vi "LSMcontroller_v62_updatedpointscan.vi"() -> ()   [LabVIEW 2015] (continued)
                n4196 = call "waveformsDObuffer.vi"("DO wf in"=w1149, "command"="set") -> ()  [unwired: 1 out]
                n4197 = call "waveformsAObuffer.vi"("AO wf in"=w1151, "command"="set") -> ()  [unwired: 1 out]
                n4198 = local write "Total Camera Frames"(w1150) -> ()
                n4199 = case shown="True" w1147 {
                  tunnel: w1146 -> [_ w1160]
                  frame False {
                  }
                  frame True {
                    n4200 = local write "# of frames"(w1160) -> ()
                  }
                }
              }
              frame #3 {
                n4201 = local read "finite samples"() -> (w1161:bool)
                n4202 = local read "continuous"() -> (w1162:bool)
                n4203 = local read "wavdet"() -> (w1163:bool)
                n4204 = call "2pparameters.vi"("command"="get") -> ("params out"=w1166:T10)  [unwired: 1 in]
                n4205 = Bundle By Name(cluster=w1166, "finite"=w1161, "cont"=w1162, "wavdet"=w1163) -> (w1164:T10)
                n4206 = call "2pparameters.vi"("Params in"=w1164, "command"="set") -> ()  [unwired: 1 out]
              }
            }
          }
          event "Start amplitude (V)", "Cycles", "Baseline (V)", "Step size (V)", "DC (%)", "Period (ms)", "Repeats", "Pulses", "phase shift (ms)": Value Change {
            n4207 = event-data() -> ()  [unwired: 1 in, 6 out]
            n4208 = stacked-sequence {
              seq-local: [_ _ w1274 _ _] -> [_ _ _ w1296 _]
              seq-local: [_ _ w1273 _ _] -> [_ _ _ w1295 _]
              frame #0 {
                n4209 = local read "Measurement"() -> (w1168:T4)
                n4210 = case shown="\"X-Y-t movie\", Default" w1168 {
                  frame "X-Y-t movie", Default {
                    n4211 = local read "avpp"() -> (w1189:i32)
                    n4212 = local read "Angle ref"() -> (w1188:dbl)
                    n4213 = local read "ROI Type"() -> (w1187:u16)
                    n4214 = local read "xpixels ref"() -> (w1184:i32)
                    n4215 = local read "Vx-min ref"() -> (w1183:dbl)
                    n4216 = local read "Vx-max ref"() -> (w1182:dbl)
                    n4217 = local read "ypixels ref"() -> (w1180:i32)
                    n4218 = local read "Vy-min ref"() -> (w1181:dbl)
                    n4219 = local read "Vy-max ref"() -> (w1177:dbl)
                    n4220 = local read "Sampling rate"() -> (w1171:dbl)
                    n4221 = local read "finite samples"() -> (w1172:bool)
                    n4222 = local read "continuous"() -> (w1175:bool)
                    n4223 = local read "wavdet"() -> (w1176:bool)
                    n4224 = local read "# of frames"() -> (w1174:i32)
                    n4225 = local read "maxbufferAI"() -> (w1173:i32)
                    n4226 = local read "Override AI buffer"() -> (w1169:bool)
                    n4227 = call "2pparameters.vi"("command"="get") -> ("params out"=w1186:T10)  [unwired: 1 in]
                    n4228 = Bundle By Name(cluster=w1186, "type"="X-Y-t movie", "avpp"=w1189, "Angle Img"=w1188, "Xpixels Img"=w1184, "Vx-min Img"=w1183, "VX-max Img"=w1182, "Ypixels Img"=w1180, "Vy-min Img"=w1181, "Vy-max Img"=w1177, "srate"=w1171, "srate Img"=w1171, "finite"=w1172, "cont"=w1175, "wavdet"=w1176, "measpoints"=w1174, "maxbufferAI"=w1173, "Drawing Mode"=w1187, "Vz-reset"=0.0, "AIoverride"=w1169) -> (w1178:T10)
                    n4229 = call "2pparameters.vi"("Params in"=w1178, "command"="set") -> ()  [unwired: 1 out]
                  }
                  frame "X-Y-Z stack" {
                    n4230 = call "2pparameters.vi"("command"="get") -> ("params out"=w1193:T10)  [unwired: 1 in]
                    n4231 = Bundle By Name(cluster=w1193, "type"="X-Y-Z stack") -> (w1191:T10)
                    n4232 = call "2pparameters.vi"("Params in"=w1191, "command"="set") -> ()  [unwired: 1 out]
                  }
                  frame "Lifetime (scan)" {
                    n4233 = call "2pparameters.vi"("command"="get") -> ("params out"=w1198:T10)  [unwired: 1 in]
                    n4234 = Bundle By Name(cluster=w1198, "type"="Lifetime (scan)") -> (w1196:T10)
                    n4235 = call "2pparameters.vi"("Params in"=w1196, "command"="set") -> ()  [unwired: 1 out]
                  }
                  frame "Lifetime (contour)" {
                    n4236 = local read "Vy-min draw"() -> (w1208:dbl)
                    n4237 = local read "Vy-max draw"() -> (w1207:dbl)
                    n4238 = local read "Vx-min draw"() -> (w1210:dbl)
                    n4239 = local read "Vx-max draw"() -> (w1209:dbl)
                    n4240 = local read "xpixels ref"() -> (w1206:i32)
                    n4241 = local read "ypixels ref"() -> (w1205:i32)
                    n4242 = local read "ROI Type"() -> (w1204:u16)
                    n4243 = local read "srateAODOtt"() -> (w1215:dbl)
                    n4244 = local read "# of frames"() -> (w1220:i32)
                    n4245 = local read "refreshtime"() -> (w1212:dbl)
                    n4246 = local read "Pel"() -> (w1203:dbl)
                    n4247 = local read "bin"() -> (w1218:dbl)
                    n4248 = local read "Override AI buffer"() -> (w1201:bool)
                    n4249 = local read "finite samples"() -> (w1227:bool)
                    n4250 = local read "srateAODOtt"() -> (w1214:dbl)
                    n4251 = local read "srateAODOtt"() -> (w1221:dbl)
                    n4252 = local read "continuous"() -> (w1226:bool)
                    n4253 = local read "Angle ref"() -> (w1211:dbl)
                    n4254 = local read "wavdet"() -> (w1228:bool)
                    n4255 = local read "Vx-ref"() -> (w1223:dbl)
                    n4256 = local read "Vy-ref"() -> (w1225:dbl)
                    n4257 = local read "avpp"() -> (w1224:i32)
                    n4258 = call "tt_timeandsamples.vi"("bin"=w1218, "refreshtime"=w1212, "srateAODOtt"=w1215, "tot#ofsamples"=w1220) -> ("refreshrate"=w1216:dbl, "refreshbuffer"=w1217:i32, "timetracecycles"=w1222:i32)  [unwired: 5 in]
                    n4259 = local read "bin"() -> (w1219:dbl)
                    n4260 = call "2pparameters.vi"("command"="get") -> ("params out"=w1231:T10)  [unwired: 1 in]
                    n4261 = Bundle By Name(cluster=w1231, "Drawing Mode"=w1204, "measpoints"=w1220, "tt_cycles"=w1222, "refreshbuffer"=w1217, "refreshrate"=w1216, "Vx-ref"=w1223, "Vy-ref"=w1225, "srate"=w1214, "finite"=w1227, "cont"=w1226, "wavdet"=w1228, "avpp"=w1224, "srateAODO"=w1221, "bufferAI"=w1217, "bin"=w1219, "Angle Img"=w1211, "Vxminref"=w1210, "Vxmaxref"=w1209, "Vyminref"=w1208, "Vymaxref"=w1207, "Xpixels Img"=w1206, "Ypixels Img"=w1205, "Pel"=w1203, "Vz-reset"=0.0, "AIoverride"=w1201, "type"="Lifetime (contour)") -> (w1229:T10)
                    n4262 = Reciprocal(x=w1216) -> (1/x=w1213:dbl)
                    n4263 = local write "refreshtime"(w1213) -> ()
                    n4264 = call "2pparameters.vi"("Params in"=w1229, "command"="set") -> ()  [unwired: 1 out]
                  }
                  frame "X-Y-Z-t movie" {
                  }
                  frame "linescan" {
                  }
                  frame "Timetrace" {
                    n4265 = local read "Vy-min draw"() -> (w1241:dbl)
                    n4266 = local read "Vy-max draw"() -> (w1240:dbl)
                    n4267 = local read "Vx-min draw"() -> (w1243:dbl)
                    n4268 = local read "Vx-max draw"() -> (w1242:dbl)
                    n4269 = local read "xpixels ref"() -> (w1239:i32)
                    n4270 = local read "ypixels ref"() -> (w1238:i32)
                    n4271 = local read "ROI Type"() -> (w1237:u16)
                    n4272 = local read "srateAODOtt"() -> (w1248:dbl)
                    n4273 = local read "# of frames"() -> (w1253:i32)
                    n4274 = local read "refreshtime"() -> (w1245:dbl)
                    n4275 = local read "Pel"() -> (w1236:dbl)
                    n4276 = local read "bin"() -> (w1251:dbl)
                    n4277 = local read "Override AI buffer"() -> (w1234:bool)
                    n4278 = local read "finite samples"() -> (w1260:bool)
                    n4279 = local read "srateAODOtt"() -> (w1247:dbl)
                    n4280 = local read "srateAODOtt"() -> (w1254:dbl)
                    n4281 = local read "continuous"() -> (w1259:bool)
                    n4282 = local read "Angle ref"() -> (w1244:dbl)
                    n4283 = local read "wavdet"() -> (w1261:bool)
                    n4284 = local read "Vx-ref"() -> (w1256:dbl)
                    n4285 = local read "Vy-ref"() -> (w1258:dbl)
                    n4286 = local read "avpp"() -> (w1257:i32)
                    n4287 = call "tt_timeandsamples.vi"("bin"=w1251, "refreshtime"=w1245, "srateAODOtt"=w1248, "tot#ofsamples"=w1253) -> ("refreshrate"=w1249:dbl, "refreshbuffer"=w1250:i32, "timetracecycles"=w1255:i32)  [unwired: 5 in]
                    n4288 = local read "bin"() -> (w1252:dbl)
                    n4289 = call "2pparameters.vi"("command"="get") -> ("params out"=w1264:T10)  [unwired: 1 in]
                    n4290 = Bundle By Name(cluster=w1264, "Drawing Mode"=w1237, "measpoints"=w1253, "tt_cycles"=w1255, "refreshbuffer"=w1250, "refreshrate"=w1249, "Vx-ref"=w1256, "Vy-ref"=w1258, "srate"=w1247, "finite"=w1260, "cont"=w1259, "wavdet"=w1261, "avpp"=w1257, "srateAODO"=w1254, "bufferAI"=w1250, "bin"=w1252, "Angle Img"=w1244, "Vxminref"=w1243, "Vxmaxref"=w1242, "Vyminref"=w1241, "Vymaxref"=w1240, "Xpixels Img"=w1239, "Ypixels Img"=w1238, "Pel"=w1236, "Vz-reset"=0.0, "AIoverride"=w1234, "type"="Timetrace") -> (w1262:T10)
                    n4291 = Reciprocal(x=w1249) -> (1/x=w1246:dbl)
                    n4292 = local write "refreshtime"(w1246) -> ()
                    n4293 = call "2pparameters.vi"("Params in"=w1262, "command"="set") -> ()  [unwired: 1 out]
                  }
                  frame "Lifetime (point)" {
                  }
                }
              }
              frame #1 {
                w1267 = FALSE ("wavdet")
                n4294 = call "2pparameters.vi"("command"="get") -> ("params out"=w1271:T10)  [unwired: 1 in]
                n4295 = Bundle By Name(cluster=w1271, "finite"=w1267, "cont"=w1267, "wavdet"=TRUE) -> (w1268:T10)
                n4296 = call "2pparameters.vi"("Params in"=w1268, "command"="set") -> ()  [unwired: 1 out]
              }
              frame #2 {
                n4297 = local read "AO channels"() -> (w1276:u32)
                n4298 = call "2pparameters.vi"("command"="get") -> ("params out"=w1278:T10)  [unwired: 1 in]
                n4299 = Unbundle By Name(w1278) -> ("aAO"=w1277:u32[])
                n4300 = Search 1D Array(1D array=w1277, element=w1276) -> (index of element=w1274:i32)  [unwired: 1 in]
                n4301 = Greater?(x=w1274, y=-1) -> (0:w1273:bool)
                n4302 = case shown="True" w1273 {
                  tunnel: w1274 -> [_ w1292]
                  frame False {
                  }
                  frame True {
                    n4303 = local read "Meastab"() -> (w1281:enum32{"X-Y Image", "Linescan", "Timetrace"})
                    n4304 = case shown="\"Timetrace\"" w1281 {
                      tunnel: [w1293 w1294] -> w1280
                      frame "X-Y Image", Default {
                        n4305 = local read "Sampling rate"() -> (w1293:dbl)
                      }
                      frame "Timetrace" {
                        n4306 = local read "srateAODOtt"() -> (w1294:dbl)
                      }
                    }
                    n4307 = local read "Start amplitude (V)"() -> (w1289:dbl)
                    n4308 = local read "phase shift (ms)"() -> (w1284:dbl)
                    n4309 = local read "Step size (V)"() -> (w1287:dbl)
                    n4310 = local read "Baseline (V)"() -> (w1288:dbl)
                    n4311 = local read "Period (ms)"() -> (w1285:dbl)
                    n4312 = local read "padding value"() -> (w1282:dbl)
                    n4313 = local read "Repeats"() -> (w1291:dbl)
                    n4314 = local read "Cycles"() -> (w1290:dbl)
                    n4315 = local read "DC (%)"() -> (w1286:dbl)
                    n4316 = local read "Pulses"() -> (w1283:dbl)
                    n4317 = call "replace AO square wf param.vi"("Baseline (V)"=w1288, "Start amplitude (V)"=w1289, "Cycles"=w1290, "Repeats"=w1291, "index of AO wave"=w1292, "Step size (V)"=w1287, "DC (%)"=w1286, "Sampling frequency (Hz)"=w1280, "Period (ms)"=w1285, "Cycle length (s)"=w1284, "Pulses"=w1283, "padding value"=w1282) -> ()  [unwired: 4 in]
                  }
                }
              }
              frame #3 {
                n4318 = case shown="True" w1295 {
                  tunnel: w1296 -> [_ w1304]
                  frame False {
                  }
                  frame True {
                    n4319 = call "waveformparamsv2.vi"("command"="get") -> ("Params out"=w1318:T14)  [unwired: 4 in, 2 out]
                    n4320 = Unbundle By Name(w1318) -> ("AO parameters"=w1317:T15)
                    n4321 = local read "Meastab"() -> (w1299:enum32{"X-Y Image", "Linescan", "Timetrace"})
                    n4322 = case shown="\"Timetrace\"" w1299 {
                      tunnel: [w1320 w1321] -> w1308
                      frame "X-Y Image", Default {
                        n4323 = local read "Sampling rate"() -> (w1320:dbl)
                      }
                      frame "Timetrace" {
                        n4324 = local read "srateAODOtt"() -> (w1321:dbl)
                      }
                    }
                    n4325 = Index Array(array=w1317, index=w1304) -> (element=w1306:T16)
                    n4326 = call "waveformsAObuffer.vi"("command"="get") -> ("AO wf out"=w1305:waveform(dbl)[])  [unwired: 1 in]
                    n4327 = call "generateRampedSquareWave_fromAOparameters.vi"("AO params"=w1306) -> ("Waveform"=w1303:waveform(dbl))  [unwired: 1 out]
                    n4328 = property on="refwf" class="Ring (strict)"() -> ("RingText.Text"=w1307:string)  [unwired: 2 in, 2 out]
                    n4329 = Replace Array Subset(array=w1305, new element=w1303, index=w1304) -> (w1302:waveform(dbl)[])
                    n4330 = call "waveformsDObuffer.vi"("command"="get") -> ("DO wf out"=w1313:digitalwaveform[])  [unwired: 1 in]
                    n4331 = call "correctwaveformsizetemp.vi"("new sampling frequency (Hz)"=w1308, "start"=FALSE, "reference waveforms to"=w1307, "Analog waveforms in"=w1302, "stop"=FALSE, "Digital waveforms in"=w1313) -> ("analog wf out"=w1311:waveform(dbl)[], "Digital wf out"=w1309:digitalwaveform[], "measpoints"=w1300:i32)
                    n4332 = local read "wavdet"() -> (w1301:bool)
                    n4333 = local write "Analog Lines Plot"(w1311) -> ()
                    n4334 = call "GetNumCamFramesv2.vi"("Digital Waveform Graph"=w1309) -> ("Numeric"=w1310:i32)  [unwired: 10 in]
                    n4335 = local write "Digital Lines Plot"(w1309) -> ()
                    n4336 = call "waveformsAObuffer.vi"("AO wf in"=w1311, "command"="set") -> ()  [unwired: 1 out]
                    n4337 = call "waveformsDObuffer.vi"("DO wf in"=w1309, "command"="set") -> ()  [unwired: 1 out]
                    n4338 = local write "Total Camera Frames"(w1310) -> ()
                    n4339 = case shown="True" w1301 {
                      tunnel: w1300 -> [_ w1322]
                      frame False {
                      }
                      frame True {
                        n4340 = local write "# of frames"(w1322) -> ()
                      }
                    }
                  }
                }
              }
              frame #4 {
                n4341 = local read "finite samples"() -> (w1323:bool)
                n4342 = local read "continuous"() -> (w1324:bool)
                n4343 = local read "wavdet"() -> (w1325:bool)
                n4344 = call "2pparameters.vi"("command"="get") -> ("params out"=w1328:T10)  [unwired: 1 in]
                n4345 = Bundle By Name(cluster=w1328, "finite"=w1323, "cont"=w1324, "wavdet"=w1325) -> (w1326:T10)
                n4346 = call "2pparameters.vi"("Params in"=w1326, "command"="set") -> ()  [unwired: 1 out]
              }
            }
          }
          event "Amplitude (V)", "Offset (V)", "Frequency", "Tri Repeats": Value Change {
            n4347 = event-data() -> ()  [unwired: 1 in, 6 out]
            n4348 = stacked-sequence {
              seq-local: [_ _ w1436 _ _] -> [_ _ _ w1454 _]
              seq-local: [_ _ w1435 _ _] -> [_ _ _ w1453 _]
              frame #0 {
                n4349 = local read "Measurement"() -> (w1330:T4)
                n4350 = case shown="\"X-Y-t movie\", Default" w1330 {
                  frame "X-Y-t movie", Default {
                    n4351 = local read "avpp"() -> (w1351:i32)
                    n4352 = local read "Angle ref"() -> (w1350:dbl)
                    n4353 = local read "ROI Type"() -> (w1349:u16)
                    n4354 = local read "xpixels ref"() -> (w1346:i32)
                    n4355 = local read "Vx-min ref"() -> (w1345:dbl)
                    n4356 = local read "Vx-max ref"() -> (w1344:dbl)
                    n4357 = local read "ypixels ref"() -> (w1342:i32)
                    n4358 = local read "Vy-min ref"() -> (w1343:dbl)
                    n4359 = local read "Vy-max ref"() -> (w1339:dbl)
                    n4360 = local read "Sampling rate"() -> (w1333:dbl)
                    n4361 = local read "finite samples"() -> (w1334:bool)
                    n4362 = local read "continuous"() -> (w1337:bool)
                    n4363 = local read "wavdet"() -> (w1338:bool)
                    n4364 = local read "# of frames"() -> (w1336:i32)
                    n4365 = local read "maxbufferAI"() -> (w1335:i32)
                    n4366 = local read "Override AI buffer"() -> (w1331:bool)
                    n4367 = call "2pparameters.vi"("command"="get") -> ("params out"=w1348:T10)  [unwired: 1 in]
                    n4368 = Bundle By Name(cluster=w1348, "type"="X-Y-t movie", "avpp"=w1351, "Angle Img"=w1350, "Xpixels Img"=w1346, "Vx-min Img"=w1345, "VX-max Img"=w1344, "Ypixels Img"=w1342, "Vy-min Img"=w1343, "Vy-max Img"=w1339, "srate"=w1333, "srate Img"=w1333, "finite"=w1334, "cont"=w1337, "wavdet"=w1338, "measpoints"=w1336, "maxbufferAI"=w1335, "Drawing Mode"=w1349, "Vz-reset"=0.0, "AIoverride"=w1331) -> (w1340:T10)
                    n4369 = call "2pparameters.vi"("Params in"=w1340, "command"="set") -> ()  [unwired: 1 out]
                  }
                  frame "X-Y-Z stack" {
                    n4370 = call "2pparameters.vi"("command"="get") -> ("params out"=w1355:T10)  [unwired: 1 in]
                    n4371 = Bundle By Name(cluster=w1355, "type"="X-Y-Z stack") -> (w1353:T10)
                    n4372 = call "2pparameters.vi"("Params in"=w1353, "command"="set") -> ()  [unwired: 1 out]
                  }
                  frame "Lifetime (scan)" {
                    n4373 = call "2pparameters.vi"("command"="get") -> ("params out"=w1360:T10)  [unwired: 1 in]
                    n4374 = Bundle By Name(cluster=w1360, "type"="Lifetime (scan)") -> (w1358:T10)
                    n4375 = call "2pparameters.vi"("Params in"=w1358, "command"="set") -> ()  [unwired: 1 out]
                  }
                  frame "Lifetime (contour)" {
                    n4376 = local read "Vy-min draw"() -> (w1370:dbl)
                    n4377 = local read "Vy-max draw"() -> (w1369:dbl)
                    n4378 = local read "Vx-min draw"() -> (w1372:dbl)
                    n4379 = local read "Vx-max draw"() -> (w1371:dbl)
                    n4380 = local read "xpixels ref"() -> (w1368:i32)
                    n4381 = local read "ypixels ref"() -> (w1367:i32)
                    n4382 = local read "ROI Type"() -> (w1366:u16)
                    n4383 = local read "srateAODOtt"() -> (w1377:dbl)
                    n4384 = local read "# of frames"() -> (w1382:i32)
                    n4385 = local read "refreshtime"() -> (w1374:dbl)
                    n4386 = local read "Pel"() -> (w1365:dbl)
                    n4387 = local read "bin"() -> (w1380:dbl)
                    n4388 = local read "Override AI buffer"() -> (w1363:bool)
                    n4389 = local read "finite samples"() -> (w1389:bool)
                    n4390 = local read "srateAODOtt"() -> (w1376:dbl)
                    n4391 = local read "srateAODOtt"() -> (w1383:dbl)
                    n4392 = local read "continuous"() -> (w1388:bool)
                    n4393 = local read "Angle ref"() -> (w1373:dbl)
                    n4394 = local read "wavdet"() -> (w1390:bool)
                    n4395 = local read "Vx-ref"() -> (w1385:dbl)
                    n4396 = local read "Vy-ref"() -> (w1387:dbl)
                    n4397 = local read "avpp"() -> (w1386:i32)
                    n4398 = call "tt_timeandsamples.vi"("bin"=w1380, "refreshtime"=w1374, "srateAODOtt"=w1377, "tot#ofsamples"=w1382) -> ("refreshrate"=w1378:dbl, "refreshbuffer"=w1379:i32, "timetracecycles"=w1384:i32)  [unwired: 5 in]
                    n4399 = local read "bin"() -> (w1381:dbl)
                    n4400 = call "2pparameters.vi"("command"="get") -> ("params out"=w1393:T10)  [unwired: 1 in]
                    n4401 = Bundle By Name(cluster=w1393, "Drawing Mode"=w1366, "measpoints"=w1382, "tt_cycles"=w1384, "refreshbuffer"=w1379, "refreshrate"=w1378, "Vx-ref"=w1385, "Vy-ref"=w1387, "srate"=w1376, "finite"=w1389, "cont"=w1388, "wavdet"=w1390, "avpp"=w1386, "srateAODO"=w1383, "bufferAI"=w1379, "bin"=w1381, "Angle Img"=w1373, "Vxminref"=w1372, "Vxmaxref"=w1371, "Vyminref"=w1370, "Vymaxref"=w1369, "Xpixels Img"=w1368, "Ypixels Img"=w1367, "Pel"=w1365, "Vz-reset"=0.0, "AIoverride"=w1363, "type"="Lifetime (contour)") -> (w1391:T10)
                    n4402 = Reciprocal(x=w1378) -> (1/x=w1375:dbl)
                    n4403 = local write "refreshtime"(w1375) -> ()
                    n4404 = call "2pparameters.vi"("Params in"=w1391, "command"="set") -> ()  [unwired: 1 out]
                  }
                  frame "X-Y-Z-t movie" {
                  }
                  frame "linescan" {
                  }
                  frame "Timetrace" {
                    n4405 = local read "Vy-min draw"() -> (w1403:dbl)
                    n4406 = local read "Vy-max draw"() -> (w1402:dbl)
                    n4407 = local read "Vx-min draw"() -> (w1405:dbl)
                    n4408 = local read "Vx-max draw"() -> (w1404:dbl)
                    n4409 = local read "xpixels ref"() -> (w1401:i32)
                    n4410 = local read "ypixels ref"() -> (w1400:i32)
                    n4411 = local read "ROI Type"() -> (w1399:u16)
                    n4412 = local read "srateAODOtt"() -> (w1410:dbl)
                    n4413 = local read "# of frames"() -> (w1415:i32)
                    n4414 = local read "refreshtime"() -> (w1407:dbl)
                    n4415 = local read "Pel"() -> (w1398:dbl)
                    n4416 = local read "bin"() -> (w1413:dbl)
                    n4417 = local read "Override AI buffer"() -> (w1396:bool)
                    n4418 = local read "finite samples"() -> (w1422:bool)
                    n4419 = local read "srateAODOtt"() -> (w1409:dbl)
                    n4420 = local read "srateAODOtt"() -> (w1416:dbl)
                    n4421 = local read "continuous"() -> (w1421:bool)
                    n4422 = local read "Angle ref"() -> (w1406:dbl)
                    n4423 = local read "wavdet"() -> (w1423:bool)
                    n4424 = local read "Vx-ref"() -> (w1418:dbl)
                    n4425 = local read "Vy-ref"() -> (w1420:dbl)
                    n4426 = local read "avpp"() -> (w1419:i32)
                    n4427 = call "tt_timeandsamples.vi"("bin"=w1413, "refreshtime"=w1407, "srateAODOtt"=w1410, "tot#ofsamples"=w1415) -> ("refreshrate"=w1411:dbl, "refreshbuffer"=w1412:i32, "timetracecycles"=w1417:i32)  [unwired: 5 in]
                    n4428 = local read "bin"() -> (w1414:dbl)
                    n4429 = call "2pparameters.vi"("command"="get") -> ("params out"=w1426:T10)  [unwired: 1 in]
                    n4430 = Bundle By Name(cluster=w1426, "Drawing Mode"=w1399, "measpoints"=w1415, "tt_cycles"=w1417, "refreshbuffer"=w1412, "refreshrate"=w1411, "Vx-ref"=w1418, "Vy-ref"=w1420, "srate"=w1409, "finite"=w1422, "cont"=w1421, "wavdet"=w1423, "avpp"=w1419, "srateAODO"=w1416, "bufferAI"=w1412, "bin"=w1414, "Angle Img"=w1406, "Vxminref"=w1405, "Vxmaxref"=w1404, "Vyminref"=w1403, "Vymaxref"=w1402, "Xpixels Img"=w1401, "Ypixels Img"=w1400, "Pel"=w1398, "Vz-reset"=0.0, "AIoverride"=w1396, "type"="Timetrace") -> (w1424:T10)
                    n4431 = Reciprocal(x=w1411) -> (1/x=w1408:dbl)
                    n4432 = local write "refreshtime"(w1408) -> ()
                    n4433 = call "2pparameters.vi"("Params in"=w1424, "command"="set") -> ()  [unwired: 1 out]
                  }
                  frame "Lifetime (point)" {
                  }
                }
              }
              frame #1 {
                w1429 = FALSE ("wavdet")
                n4434 = call "2pparameters.vi"("command"="get") -> ("params out"=w1433:T10)  [unwired: 1 in]
                n4435 = Bundle By Name(cluster=w1433, "finite"=w1429, "cont"=w1429, "wavdet"=TRUE) -> (w1430:T10)
                n4436 = call "2pparameters.vi"("Params in"=w1430, "command"="set") -> ()  [unwired: 1 out]
              }
              frame #2 {
                n4437 = local read "AO channels"() -> (w1438:u32)
                n4438 = call "2pparameters.vi"("command"="get") -> ("params out"=w1440:T10)  [unwired: 1 in]
                n4439 = Unbundle By Name(w1440) -> ("aAO"=w1439:u32[])
                n4440 = Search 1D Array(1D array=w1439, element=w1438) -> (index of element=w1436:i32)  [unwired: 1 in]
                n4441 = Greater?(x=w1436, y=-1) -> (0:w1435:bool)
                n4442 = case shown="True" w1435 {
                  tunnel: w1436 -> [_ w1450]
                  frame False {
                  }
                  frame True {
                    n4443 = local read "Meastab"() -> (w1443:enum32{"X-Y Image", "Linescan", "Timetrace"})
                    n4444 = local read "Tri padding value"() -> (w1444:dbl)
                    n4445 = local read "Amplitude (V)"() -> (w1448:dbl)
                    n4446 = local read "Tri Phase (s)"() -> (w1445:dbl)
                    n4447 = local read "Tri Repeats"() -> (w1446:dbl)
                    n4448 = local read "Frequency"() -> (w1447:dbl)
                    n4449 = local read "Offset (V)"() -> (w1449:dbl)
                    n4450 = case shown="\"Timetrace\"" w1443 {
                      tunnel: [w1451 w1452] -> w1442
                      frame "X-Y Image", Default {
                        n4451 = local read "Sampling rate"() -> (w1451:dbl)
                      }
                      frame "Timetrace" {
                        n4452 = local read "srateAODOtt"() -> (w1452:dbl)
                      }
                    }
                    n4453 = call "replace AO tri wf param.vi"("padding value"=w1444, "index of AO wave"=w1450, "Tri phase"=w1445, "Sampling frequency (Hz)"=w1442, "Tri Repeats"=w1446, "Frequency"=w1447, "Amplitude (V)"=w1448, "Offset (V)"=w1449) -> ()
                  }
                }
              }
              frame #3 {
                n4454 = case shown="True" w1453 {
                  tunnel: w1454 -> [_ w1463]
                  frame False {
                  }
                  frame True {
                    n4455 = call "waveformparamsv2.vi"("command"="get") -> ("Params out"=w1476:T14)  [unwired: 4 in, 2 out]
                    n4456 = Unbundle By Name(w1476) -> ("AO parameters"=w1475:T15)
                    n4457 = local read "Meastab"() -> (w1458:enum32{"X-Y Image", "Linescan", "Timetrace"})
                    n4458 = case shown="\"Timetrace\"" w1458 {
                      tunnel: [w1478 w1479] -> w1457
                      frame "X-Y Image", Default {
                        n4459 = local read "Sampling rate"() -> (w1478:dbl)
                      }
                      frame "Timetrace" {
                        n4460 = local read "srateAODOtt"() -> (w1479:dbl)
                      }
                    }
                    n4461 = Index Array(array=w1475, index=w1463) -> (element=w1465:T16)
                    n4462 = call "waveformsAObuffer.vi"("command"="get") -> ("AO wf out"=w1464:waveform(dbl)[])  [unwired: 1 in]
                    n4463 = call "generateTriWave_fromAOparameters.vi"("AO params"=w1465) -> ("Waveform"=w1462:waveform(dbl))  [unwired: 1 out]
                    n4464 = property on="refwf" class="Ring (strict)"() -> ("RingText.Text"=w1466:string)  [unwired: 2 in, 2 out]
                    n4465 = Replace Array Subset(array=w1464, new element=w1462, index=w1463) -> (w1461:waveform(dbl)[])
                    n4466 = call "waveformsDObuffer.vi"("command"="get") -> ("DO wf out"=w1471:digitalwaveform[])  [unwired: 1 in]
                    n4467 = call "correctwaveformsizetemp.vi"("new sampling frequency (Hz)"=w1457, "start"=FALSE, "reference waveforms to"=w1466, "Analog waveforms in"=w1461, "stop"=FALSE, "Digital waveforms in"=w1471) -> ("analog wf out"=w1469:waveform(dbl)[], "Digital wf out"=w1467:digitalwaveform[], "measpoints"=w1459:i32)
                    n4468 = local read "wavdet"() -> (w1460:bool)
                    n4469 = local write "Analog Lines Plot"(w1469) -> ()
                    n4470 = call "GetNumCamFramesv2.vi"("Digital Waveform Graph"=w1467) -> ("Numeric"=w1468:i32)  [unwired: 10 in]
                    n4471 = local write "Digital Lines Plot"(w1467) -> ()
                    n4472 = call "waveformsAObuffer.vi"("AO wf in"=w1469, "command"="set") -> ()  [unwired: 1 out]
                    n4473 = call "waveformsDObuffer.vi"("DO wf in"=w1467, "command"="set") -> ()  [unwired: 1 out]
                    n4474 = local write "Total Camera Frames"(w1468) -> ()
                    n4475 = case shown="True" w1460 {
                      tunnel: w1459 -> [_ w1480]
                      frame False {
                      }
                      frame True {
                        n4476 = local write "# of frames"(w1480) -> ()
                      }
                    }
                  }
                }
              }
              frame #4 {
                n4477 = local read "finite samples"() -> (w1481:bool)
                n4478 = local read "continuous"() -> (w1482:bool)
                n4479 = local read "wavdet"() -> (w1483:bool)
                n4480 = call "2pparameters.vi"("command"="get") -> ("params out"=w1486:T10)  [unwired: 1 in]
                n4481 = Bundle By Name(cluster=w1486, "finite"=w1481, "cont"=w1482, "wavdet"=w1483) -> (w1484:T10)
                n4482 = call "2pparameters.vi"("Params in"=w1484, "command"="set") -> ()  [unwired: 1 out]
              }
            }
          }
          event "Load Matlab Waveform": Value Change {
            n4483 = event-data() -> ()  [unwired: 1 in, 6 out]
            n4484 = stacked-sequence {
              seq-local: [_ _ w1594 _ _] -> [_ _ _ w1609 _]
              seq-local: [_ _ w1593 _ _] -> [_ _ _ w1608 _]
              frame #0 {
                n4485 = local read "Measurement"() -> (w1488:T4)
                n4486 = case shown="\"X-Y-t movie\", Default" w1488 {
                  frame "X-Y-t movie", Default {
                    n4487 = local read "avpp"() -> (w1509:i32)
                    n4488 = local read "Angle ref"() -> (w1508:dbl)
                    n4489 = local read "ROI Type"() -> (w1507:u16)
                    n4490 = local read "xpixels ref"() -> (w1504:i32)
                    n4491 = local read "Vx-min ref"() -> (w1503:dbl)
                    n4492 = local read "Vx-max ref"() -> (w1502:dbl)
                    n4493 = local read "ypixels ref"() -> (w1500:i32)
                    n4494 = local read "Vy-min ref"() -> (w1501:dbl)
                    n4495 = local read "Vy-max ref"() -> (w1497:dbl)
                    n4496 = local read "Sampling rate"() -> (w1491:dbl)
                    n4497 = local read "finite samples"() -> (w1492:bool)
                    n4498 = local read "continuous"() -> (w1495:bool)
                    n4499 = local read "wavdet"() -> (w1496:bool)
                    n4500 = local read "# of frames"() -> (w1494:i32)
                    n4501 = local read "maxbufferAI"() -> (w1493:i32)
                    n4502 = local read "Override AI buffer"() -> (w1489:bool)
                    n4503 = call "2pparameters.vi"("command"="get") -> ("params out"=w1506:T10)  [unwired: 1 in]
                    n4504 = Bundle By Name(cluster=w1506, "type"="X-Y-t movie", "avpp"=w1509, "Angle Img"=w1508, "Xpixels Img"=w1504, "Vx-min Img"=w1503, "VX-max Img"=w1502, "Ypixels Img"=w1500, "Vy-min Img"=w1501, "Vy-max Img"=w1497, "srate"=w1491, "srate Img"=w1491, "finite"=w1492, "cont"=w1495, "wavdet"=w1496, "measpoints"=w1494, "maxbufferAI"=w1493, "Drawing Mode"=w1507, "Vz-reset"=0.0, "AIoverride"=w1489) -> (w1498:T10)
                    n4505 = call "2pparameters.vi"("Params in"=w1498, "command"="set") -> ()  [unwired: 1 out]
                  }
                  frame "X-Y-Z stack" {
                    n4506 = call "2pparameters.vi"("command"="get") -> ("params out"=w1513:T10)  [unwired: 1 in]
                    n4507 = Bundle By Name(cluster=w1513, "type"="X-Y-Z stack") -> (w1511:T10)
                    n4508 = call "2pparameters.vi"("Params in"=w1511, "command"="set") -> ()  [unwired: 1 out]
                  }
                  frame "Lifetime (scan)" {
                    n4509 = call "2pparameters.vi"("command"="get") -> ("params out"=w1518:T10)  [unwired: 1 in]
                    n4510 = Bundle By Name(cluster=w1518, "type"="Lifetime (scan)") -> (w1516:T10)
                    n4511 = call "2pparameters.vi"("Params in"=w1516, "command"="set") -> ()  [unwired: 1 out]
                  }
                  frame "Lifetime (contour)" {
                    n4512 = local read "Vy-min draw"() -> (w1528:dbl)
                    n4513 = local read "Vy-max draw"() -> (w1527:dbl)
                    n4514 = local read "Vx-min draw"() -> (w1530:dbl)
                    n4515 = local read "Vx-max draw"() -> (w1529:dbl)
                    n4516 = local read "xpixels ref"() -> (w1526:i32)
                    n4517 = local read "ypixels ref"() -> (w1525:i32)
                    n4518 = local read "ROI Type"() -> (w1524:u16)
                    n4519 = local read "srateAODOtt"() -> (w1535:dbl)
                    n4520 = local read "# of frames"() -> (w1540:i32)
                    n4521 = local read "refreshtime"() -> (w1532:dbl)
                    n4522 = local read "Pel"() -> (w1523:dbl)
                    n4523 = local read "bin"() -> (w1538:dbl)
                    n4524 = local read "Override AI buffer"() -> (w1521:bool)
                    n4525 = local read "finite samples"() -> (w1547:bool)
                    n4526 = local read "srateAODOtt"() -> (w1534:dbl)
                    n4527 = local read "srateAODOtt"() -> (w1541:dbl)
                    n4528 = local read "continuous"() -> (w1546:bool)
                    n4529 = local read "Angle ref"() -> (w1531:dbl)
                    n4530 = local read "wavdet"() -> (w1548:bool)
                    n4531 = local read "Vx-ref"() -> (w1543:dbl)
                    n4532 = local read "Vy-ref"() -> (w1545:dbl)
                    n4533 = local read "avpp"() -> (w1544:i32)
                    n4534 = call "tt_timeandsamples.vi"("bin"=w1538, "refreshtime"=w1532, "srateAODOtt"=w1535, "tot#ofsamples"=w1540) -> ("refreshrate"=w1536:dbl, "refreshbuffer"=w1537:i32, "timetracecycles"=w1542:i32)  [unwired: 5 in]
                    n4535 = local read "bin"() -> (w1539:dbl)
                    n4536 = call "2pparameters.vi"("command"="get") -> ("params out"=w1551:T10)  [unwired: 1 in]
                    n4537 = Bundle By Name(cluster=w1551, "Drawing Mode"=w1524, "measpoints"=w1540, "tt_cycles"=w1542, "refreshbuffer"=w1537, "refreshrate"=w1536, "Vx-ref"=w1543, "Vy-ref"=w1545, "srate"=w1534, "finite"=w1547, "cont"=w1546, "wavdet"=w1548, "avpp"=w1544, "srateAODO"=w1541, "bufferAI"=w1537, "bin"=w1539, "Angle Img"=w1531, "Vxminref"=w1530, "Vxmaxref"=w1529, "Vyminref"=w1528, "Vymaxref"=w1527, "Xpixels Img"=w1526, "Ypixels Img"=w1525, "Pel"=w1523, "Vz-reset"=0.0, "AIoverride"=w1521, "type"="Lifetime (contour)") -> (w1549:T10)
                    n4538 = Reciprocal(x=w1536) -> (1/x=w1533:dbl)
                    n4539 = local write "refreshtime"(w1533) -> ()
                    n4540 = call "2pparameters.vi"("Params in"=w1549, "command"="set") -> ()  [unwired: 1 out]
                  }
                  frame "X-Y-Z-t movie" {
                  }
                  frame "linescan" {
                  }
                  frame "Timetrace" {
                    n4541 = local read "Vy-min draw"() -> (w1561:dbl)
                    n4542 = local read "Vy-max draw"() -> (w1560:dbl)
                    n4543 = local read "Vx-min draw"() -> (w1563:dbl)
                    n4544 = local read "Vx-max draw"() -> (w1562:dbl)
                    n4545 = local read "xpixels ref"() -> (w1559:i32)
                    n4546 = local read "ypixels ref"() -> (w1558:i32)
                    n4547 = local read "ROI Type"() -> (w1557:u16)
                    n4548 = local read "srateAODOtt"() -> (w1568:dbl)
                    n4549 = local read "# of frames"() -> (w1573:i32)
                    n4550 = local read "refreshtime"() -> (w1565:dbl)
                    n4551 = local read "Pel"() -> (w1556:dbl)
                    n4552 = local read "bin"() -> (w1571:dbl)
                    n4553 = local read "Override AI buffer"() -> (w1554:bool)
                    n4554 = local read "finite samples"() -> (w1580:bool)
                    n4555 = local read "srateAODOtt"() -> (w1567:dbl)
                    n4556 = local read "srateAODOtt"() -> (w1574:dbl)
                    n4557 = local read "continuous"() -> (w1579:bool)
                    n4558 = local read "Angle ref"() -> (w1564:dbl)
                    n4559 = local read "wavdet"() -> (w1581:bool)
                    n4560 = local read "Vx-ref"() -> (w1576:dbl)
                    n4561 = local read "Vy-ref"() -> (w1578:dbl)
                    n4562 = local read "avpp"() -> (w1577:i32)
                    n4563 = call "tt_timeandsamples.vi"("bin"=w1571, "refreshtime"=w1565, "srateAODOtt"=w1568, "tot#ofsamples"=w1573) -> ("refreshrate"=w1569:dbl, "refreshbuffer"=w1570:i32, "timetracecycles"=w1575:i32)  [unwired: 5 in]
                    n4564 = local read "bin"() -> (w1572:dbl)
                    n4565 = call "2pparameters.vi"("command"="get") -> ("params out"=w1584:T10)  [unwired: 1 in]
                    n4566 = Bundle By Name(cluster=w1584, "Drawing Mode"=w1557, "measpoints"=w1573, "tt_cycles"=w1575, "refreshbuffer"=w1570, "refreshrate"=w1569, "Vx-ref"=w1576, "Vy-ref"=w1578, "srate"=w1567, "finite"=w1580, "cont"=w1579, "wavdet"=w1581, "avpp"=w1577, "srateAODO"=w1574, "bufferAI"=w1570, "bin"=w1572, "Angle Img"=w1564, "Vxminref"=w1563, "Vxmaxref"=w1562, "Vyminref"=w1561, "Vymaxref"=w1560, "Xpixels Img"=w1559, "Ypixels Img"=w1558, "Pel"=w1556, "Vz-reset"=0.0, "AIoverride"=w1554, "type"="Timetrace") -> (w1582:T10)
                    n4567 = Reciprocal(x=w1569) -> (1/x=w1566:dbl)
                    n4568 = local write "refreshtime"(w1566) -> ()
                    n4569 = call "2pparameters.vi"("Params in"=w1582, "command"="set") -> ()  [unwired: 1 out]
                  }
                  frame "Lifetime (point)" {
                  }
                }
              }
              frame #1 {
                w1587 = FALSE ("wavdet")
                n4570 = call "2pparameters.vi"("command"="get") -> ("params out"=w1591:T10)  [unwired: 1 in]
                n4571 = Bundle By Name(cluster=w1591, "finite"=w1587, "cont"=w1587, "wavdet"=TRUE) -> (w1588:T10)
                n4572 = call "2pparameters.vi"("Params in"=w1588, "command"="set") -> ()  [unwired: 1 out]
              }
              frame #2 {
                n4573 = local read "AO channels"() -> (w1596:u32)
                n4574 = call "2pparameters.vi"("command"="get") -> ("params out"=w1598:T10)  [unwired: 1 in]
                n4575 = Unbundle By Name(w1598) -> ("aAO"=w1597:u32[])
                n4576 = Search 1D Array(1D array=w1597, element=w1596) -> (index of element=w1594:i32)  [unwired: 1 in]
                n4577 = Greater?(x=w1594, y=-1) -> (0:w1593:bool)
                n4578 = case shown="True" w1593 {
                  tunnel: w1594 -> [_ w1605]
                  frame False {
                  }
                  frame True {
                    n4579 = local read "Meastab"() -> (w1601:enum32{"X-Y Image", "Linescan", "Timetrace"})
                    n4580 = local read "Matlab waveform path"() -> (w1603:path)
                    n4581 = local read "Matlab padding value"() -> (w1604:dbl)
                    n4582 = case shown="\"Timetrace\"" w1601 {
                      tunnel: [w1606 w1607] -> w1600
                      frame "X-Y Image", Default {
                        n4583 = local read "Sampling rate"() -> (w1606:dbl)
                      }
                      frame "Timetrace" {
                        n4584 = local read "srateAODOtt"() -> (w1607:dbl)
                      }
                    }
                    n4585 = call "matlabwfexistsdialogue.vi"("Matlab waveform path"=w1603) -> ("mtalab waveform path out"=w1602:path)
                    n4586 = call "replace AO matlab param.vi"("Sampling frequency (Hz)"=w1600, "matlab wave file"=w1602, "index of AO wave"=w1605, "padding value"=w1604) -> ()  [unwired: 7 in]
                  }
                }
              }
              frame #3 {
                n4587 = case shown="True" w1608 {
                  tunnel: w1609 -> [_ w1616]
                  frame False {
                  }
                  frame True {
                    n4588 = local read "Meastab"() -> (w1613:enum32{"X-Y Image", "Linescan", "Timetrace"})
                    n4589 = call "waveformparamsv2.vi"("command"="get") -> ("Params out"=w1619:T14)  [unwired: 4 in, 2 out]
                    n4590 = Unbundle By Name(w1619) -> ("AO parameters"=w1618:T15)
                    n4591 = case shown="\"Timetrace\"" w1613 {
                      tunnel: [w1633 w1634] -> w1612
                      frame "X-Y Image", Default {
                        n4592 = local read "Sampling rate"() -> (w1633:dbl)
                      }
                      frame "Timetrace" {
                        n4593 = local read "srateAODOtt"() -> (w1634:dbl)
                      }
                    }
                    n4594 = Index Array(array=w1618, index=w1616) -> (element=w1617:T16)
                    n4595 = call "waveformsAObuffer.vi"("command"="get") -> ("AO wf out"=w1623:waveform(dbl)[])  [unwired: 1 in]
                    n4596 = call "matlabAOwffromparam.vi"("Cluster"=w1617) -> ("Waveform"=w1621:waveform(dbl))  [unwired: 1 out]
                    n4597 = property on="refwf" class="Ring (strict)"() -> ("RingText.Text"=w1624:string)  [unwired: 2 in, 2 out]
                    n4598 = Replace Array Subset(array=w1623, new element=w1621, index=w1616) -> (w1622:waveform(dbl)[])
                    n4599 = call "waveformsDObuffer.vi"("command"="get") -> ("DO wf out"=w1629:digitalwaveform[])  [unwired: 1 in]
                    n4600 = call "correctwaveformsizetemp.vi"("new sampling frequency (Hz)"=w1612, "start"=FALSE, "reference waveforms to"=w1624, "Analog waveforms in"=w1622, "stop"=FALSE, "Digital waveforms in"=w1629) -> ("analog wf out"=w1627:waveform(dbl)[], "Digital wf out"=w1625:digitalwaveform[], "measpoints"=w1614:i32)
                    n4601 = local read "wavdet"() -> (w1615:bool)
                    n4602 = local write "Analog Lines Plot"(w1627) -> ()
                    n4603 = call "GetNumCamFramesv2.vi"("Digital Waveform Graph"=w1625) -> ("Numeric"=w1626:i32)  [unwired: 10 in]
                    n4604 = local write "Digital Lines Plot"(w1625) -> ()
                    n4605 = call "waveformsAObuffer.vi"("AO wf in"=w1627, "command"="set") -> ()  [unwired: 1 out]
                    n4606 = call "waveformsDObuffer.vi"("DO wf in"=w1625, "command"="set") -> ()  [unwired: 1 out]
                    n4607 = local write "Total Camera Frames"(w1626) -> ()
                    n4608 = case shown="True" w1615 {
                      tunnel: w1614 -> [_ w1635]
                      frame False {
                      }
                      frame True {
                        n4609 = local write "# of frames"(w1635) -> ()
                      }
                    }
                  }
                }
              }
              frame #4 {
                n4610 = local read "finite samples"() -> (w1636:bool)
                n4611 = local read "continuous"() -> (w1637:bool)
                n4612 = local read "wavdet"() -> (w1638:bool)
                n4613 = call "2pparameters.vi"("command"="get") -> ("params out"=w1641:T10)  [unwired: 1 in]
                n4614 = Bundle By Name(cluster=w1641, "finite"=w1636, "cont"=w1637, "wavdet"=w1638) -> (w1639:T10)
                n4615 = call "2pparameters.vi"("Params in"=w1639, "command"="set") -> ()  [unwired: 1 out]
              }
            }
          }
          event "Load Matlab Waveform DO": Value Change {
            n4616 = event-data() -> ()  [unwired: 1 in, 6 out]
            n4617 = stacked-sequence {
              seq-local: [_ _ w1749 _ _] -> [_ _ _ w1764 _]
              seq-local: [_ _ w1748 _ _] -> [_ _ _ w1763 _]
              frame #0 {
                n4618 = local read "Measurement"() -> (w1643:T4)
                n4619 = case shown="\"X-Y-t movie\", Default" w1643 {
                  frame "X-Y-t movie", Default {
                    n4620 = local read "avpp"() -> (w1664:i32)
                    n4621 = local read "Angle ref"() -> (w1663:dbl)
                    n4622 = local read "ROI Type"() -> (w1662:u16)
                    n4623 = local read "xpixels ref"() -> (w1659:i32)
                    n4624 = local read "Vx-min ref"() -> (w1658:dbl)
                    n4625 = local read "Vx-max ref"() -> (w1657:dbl)
                    n4626 = local read "ypixels ref"() -> (w1655:i32)
                    n4627 = local read "Vy-min ref"() -> (w1656:dbl)
                    n4628 = local read "Vy-max ref"() -> (w1652:dbl)
                    n4629 = local read "Sampling rate"() -> (w1646:dbl)
                    n4630 = local read "finite samples"() -> (w1647:bool)
                    n4631 = local read "continuous"() -> (w1650:bool)
                    n4632 = local read "wavdet"() -> (w1651:bool)
                    n4633 = local read "# of frames"() -> (w1649:i32)
                    n4634 = local read "maxbufferAI"() -> (w1648:i32)
                    n4635 = local read "Override AI buffer"() -> (w1644:bool)
                    n4636 = call "2pparameters.vi"("command"="get") -> ("params out"=w1661:T10)  [unwired: 1 in]
                    n4637 = Bundle By Name(cluster=w1661, "type"="X-Y-t movie", "avpp"=w1664, "Angle Img"=w1663, "Xpixels Img"=w1659, "Vx-min Img"=w1658, "VX-max Img"=w1657, "Ypixels Img"=w1655, "Vy-min Img"=w1656, "Vy-max Img"=w1652, "srate"=w1646, "srate Img"=w1646, "finite"=w1647, "cont"=w1650, "wavdet"=w1651, "measpoints"=w1649, "maxbufferAI"=w1648, "Drawing Mode"=w1662, "Vz-reset"=0.0, "AIoverride"=w1644) -> (w1653:T10)
                    n4638 = call "2pparameters.vi"("Params in"=w1653, "command"="set") -> ()  [unwired: 1 out]
                  }
                  frame "X-Y-Z stack" {
                    n4639 = call "2pparameters.vi"("command"="get") -> ("params out"=w1668:T10)  [unwired: 1 in]
                    n4640 = Bundle By Name(cluster=w1668, "type"="X-Y-Z stack") -> (w1666:T10)
                    n4641 = call "2pparameters.vi"("Params in"=w1666, "command"="set") -> ()  [unwired: 1 out]
                  }
                  frame "Lifetime (scan)" {
                    n4642 = call "2pparameters.vi"("command"="get") -> ("params out"=w1673:T10)  [unwired: 1 in]
                    n4643 = Bundle By Name(cluster=w1673, "type"="Lifetime (scan)") -> (w1671:T10)
                    n4644 = call "2pparameters.vi"("Params in"=w1671, "command"="set") -> ()  [unwired: 1 out]
                  }
                  frame "Lifetime (contour)" {
                    n4645 = local read "Vy-min draw"() -> (w1683:dbl)
                    n4646 = local read "Vy-max draw"() -> (w1682:dbl)
                    n4647 = local read "Vx-min draw"() -> (w1685:dbl)
                    n4648 = local read "Vx-max draw"() -> (w1684:dbl)
                    n4649 = local read "xpixels ref"() -> (w1681:i32)
                    n4650 = local read "ypixels ref"() -> (w1680:i32)
                    n4651 = local read "ROI Type"() -> (w1679:u16)
                    n4652 = local read "srateAODOtt"() -> (w1690:dbl)
                    n4653 = local read "# of frames"() -> (w1695:i32)
                    n4654 = local read "refreshtime"() -> (w1687:dbl)
                    n4655 = local read "Pel"() -> (w1678:dbl)
                    n4656 = local read "bin"() -> (w1693:dbl)
                    n4657 = local read "Override AI buffer"() -> (w1676:bool)
                    n4658 = local read "finite samples"() -> (w1702:bool)
                    n4659 = local read "srateAODOtt"() -> (w1689:dbl)
                    n4660 = local read "srateAODOtt"() -> (w1696:dbl)
                    n4661 = local read "continuous"() -> (w1701:bool)
                    n4662 = local read "Angle ref"() -> (w1686:dbl)
                    n4663 = local read "wavdet"() -> (w1703:bool)
                    n4664 = local read "Vx-ref"() -> (w1698:dbl)
                    n4665 = local read "Vy-ref"() -> (w1700:dbl)
                    n4666 = local read "avpp"() -> (w1699:i32)
                    n4667 = call "tt_timeandsamples.vi"("bin"=w1693, "refreshtime"=w1687, "srateAODOtt"=w1690, "tot#ofsamples"=w1695) -> ("refreshrate"=w1691:dbl, "refreshbuffer"=w1692:i32, "timetracecycles"=w1697:i32)  [unwired: 5 in]
                    n4668 = local read "bin"() -> (w1694:dbl)
                    n4669 = call "2pparameters.vi"("command"="get") -> ("params out"=w1706:T10)  [unwired: 1 in]
                    n4670 = Bundle By Name(cluster=w1706, "Drawing Mode"=w1679, "measpoints"=w1695, "tt_cycles"=w1697, "refreshbuffer"=w1692, "refreshrate"=w1691, "Vx-ref"=w1698, "Vy-ref"=w1700, "srate"=w1689, "finite"=w1702, "cont"=w1701, "wavdet"=w1703, "avpp"=w1699, "srateAODO"=w1696, "bufferAI"=w1692, "bin"=w1694, "Angle Img"=w1686, "Vxminref"=w1685, "Vxmaxref"=w1684, "Vyminref"=w1683, "Vymaxref"=w1682, "Xpixels Img"=w1681, "Ypixels Img"=w1680, "Pel"=w1678, "Vz-reset"=0.0, "AIoverride"=w1676, "type"="Lifetime (contour)") -> (w1704:T10)
                    n4671 = Reciprocal(x=w1691) -> (1/x=w1688:dbl)
                    n4672 = local write "refreshtime"(w1688) -> ()
                    n4673 = call "2pparameters.vi"("Params in"=w1704, "command"="set") -> ()  [unwired: 1 out]
                  }
                  frame "X-Y-Z-t movie" {
                  }
                  frame "linescan" {
                  }
                  frame "Timetrace" {
                    n4674 = local read "Vy-min draw"() -> (w1716:dbl)
                    n4675 = local read "Vy-max draw"() -> (w1715:dbl)
                    n4676 = local read "Vx-min draw"() -> (w1718:dbl)
                    n4677 = local read "Vx-max draw"() -> (w1717:dbl)
                    n4678 = local read "xpixels ref"() -> (w1714:i32)
                    n4679 = local read "ypixels ref"() -> (w1713:i32)
                    n4680 = local read "ROI Type"() -> (w1712:u16)
                    n4681 = local read "srateAODOtt"() -> (w1723:dbl)
                    n4682 = local read "# of frames"() -> (w1728:i32)
                    n4683 = local read "refreshtime"() -> (w1720:dbl)
                    n4684 = local read "Pel"() -> (w1711:dbl)
                    n4685 = local read "bin"() -> (w1726:dbl)
                    n4686 = local read "Override AI buffer"() -> (w1709:bool)
                    n4687 = local read "finite samples"() -> (w1735:bool)
                    n4688 = local read "srateAODOtt"() -> (w1722:dbl)
                    n4689 = local read "srateAODOtt"() -> (w1729:dbl)
                    n4690 = local read "continuous"() -> (w1734:bool)
                    n4691 = local read "Angle ref"() -> (w1719:dbl)
                    n4692 = local read "wavdet"() -> (w1736:bool)
                    n4693 = local read "Vx-ref"() -> (w1731:dbl)
                    n4694 = local read "Vy-ref"() -> (w1733:dbl)
                    n4695 = local read "avpp"() -> (w1732:i32)
                    n4696 = call "tt_timeandsamples.vi"("bin"=w1726, "refreshtime"=w1720, "srateAODOtt"=w1723, "tot#ofsamples"=w1728) -> ("refreshrate"=w1724:dbl, "refreshbuffer"=w1725:i32, "timetracecycles"=w1730:i32)  [unwired: 5 in]
                    n4697 = local read "bin"() -> (w1727:dbl)
                    n4698 = call "2pparameters.vi"("command"="get") -> ("params out"=w1739:T10)  [unwired: 1 in]
                    n4699 = Bundle By Name(cluster=w1739, "Drawing Mode"=w1712, "measpoints"=w1728, "tt_cycles"=w1730, "refreshbuffer"=w1725, "refreshrate"=w1724, "Vx-ref"=w1731, "Vy-ref"=w1733, "srate"=w1722, "finite"=w1735, "cont"=w1734, "wavdet"=w1736, "avpp"=w1732, "srateAODO"=w1729, "bufferAI"=w1725, "bin"=w1727, "Angle Img"=w1719, "Vxminref"=w1718, "Vxmaxref"=w1717, "Vyminref"=w1716, "Vymaxref"=w1715, "Xpixels Img"=w1714, "Ypixels Img"=w1713, "Pel"=w1711, "Vz-reset"=0.0, "AIoverride"=w1709, "type"="Timetrace") -> (w1737:T10)
                    n4700 = Reciprocal(x=w1724) -> (1/x=w1721:dbl)
                    n4701 = local write "refreshtime"(w1721) -> ()
                    n4702 = call "2pparameters.vi"("Params in"=w1737, "command"="set") -> ()  [unwired: 1 out]
                  }
                  frame "Lifetime (point)" {
                  }
                }
              }
              frame #1 {
                w1742 = FALSE ("wavdet")
                n4703 = call "2pparameters.vi"("command"="get") -> ("params out"=w1746:T10)  [unwired: 1 in]
                n4704 = Bundle By Name(cluster=w1746, "finite"=w1742, "cont"=w1742, "wavdet"=TRUE) -> (w1743:T10)
                n4705 = call "2pparameters.vi"("Params in"=w1743, "command"="set") -> ()  [unwired: 1 out]
              }
              frame #2 {
                n4706 = local read "DO channels"() -> (w1751:u16)
                n4707 = call "2pparameters.vi"("command"="get") -> ("params out"=w1753:T10)  [unwired: 1 in]
                n4708 = Unbundle By Name(w1753) -> ("aDO"=w1752:u32[])
                n4709 = Search 1D Array(1D array=w1752, element=w1751) -> (index of element=w1749:i32)  [unwired: 1 in]
                n4710 = Greater?(x=w1749, y=-1) -> (0:w1748:bool)
                n4711 = case shown="True" w1748 {
                  tunnel: w1749 -> [_ w1760]
                  frame False {
                  }
                  frame True {
                    n4712 = local read "Meastab"() -> (w1756:enum32{"X-Y Image", "Linescan", "Timetrace"})
                    n4713 = local read "Matlab waveform path DO"() -> (w1758:path)
                    n4714 = local read "Matlab padding value DO"() -> (w1759:dbl)
                    n4715 = case shown="\"Timetrace\"" w1756 {
                      tunnel: [w1761 w1762] -> w1755
                      frame "X-Y Image", Default {
                        n4716 = local read "Sampling rate"() -> (w1761:dbl)
                      }
                      frame "Timetrace" {
                        n4717 = local read "srateAODOtt"() -> (w1762:dbl)
                      }
                    }
                    n4718 = call "matlabwfexistsdialogue.vi"("Matlab waveform path"=w1758) -> ("mtalab waveform path out"=w1757:path)
                    n4719 = call "replace DO matlab param.vi"("Sampling frequency (Hz)"=w1755, "matlab wave number"=w1757, "index of DO wave"=w1760, "padding value"=w1759) -> ()  [unwired: 7 in]
                  }
                }
              }
              frame #3 {
                n4720 = case shown="True" w1763 {
                  tunnel: w1764 -> [_ w1773]
                  frame False {
                  }
                  frame True {
                    n4721 = local read "Meastab"() -> (w1768:enum32{"X-Y Image", "Linescan", "Timetrace"})
                    n4722 = call "waveformparamsv2.vi"("command"="get") -> ("Params out"=w1786:T14)  [unwired: 4 in, 2 out]
                    n4723 = Unbundle By Name(w1786) -> ("DO parameters"=w1785:T17)
                    n4724 = case shown="\"Timetrace\"" w1768 {
                      tunnel: [w1788 w1789] -> w1767
                      frame "X-Y Image", Default {
                        n4725 = local read "Sampling rate"() -> (w1788:dbl)
                      }
                      frame "Timetrace" {
                        n4726 = local read "srateAODOtt"() -> (w1789:dbl)
                      }
                    }
                    n4727 = Index Array(array=w1785, index=w1773) -> (element=w1772:T18)
                    n4728 = call "waveformsDObuffer.vi"("command"="get") -> ("DO wf out"=w1783:digitalwaveform[])  [unwired: 1 in]
                    n4729 = property on="refwf" class="Ring (strict)"() -> ("RingText.Text"=w1775:string)  [unwired: 2 in, 2 out]
                    n4730 = call "matlabDOwffromparam.vi"("waveform params"=w1772) -> ("digital waveform"=w1771:digitalwaveform)
                    n4731 = Replace Array Subset(array=w1783, new element=w1771, index=w1773) -> (w1774:digitalwaveform[])
                    n4732 = call "waveformsAObuffer.vi"("command"="get") -> ("AO wf out"=w1782:waveform(dbl)[])  [unwired: 1 in]
                    n4733 = local read "wavdet"() -> (w1770:bool)
                    n4734 = call "correctwaveformsizetemp.vi"("new sampling frequency (Hz)"=w1767, "start"=FALSE, "reference waveforms to"=w1775, "Analog waveforms in"=w1782, "stop"=FALSE, "Digital waveforms in"=w1774) -> ("analog wf out"=w1778:waveform(dbl)[], "Digital wf out"=w1776:digitalwaveform[], "measpoints"=w1769:i32)
                    n4735 = local write "Analog Lines Plot"(w1778) -> ()
                    n4736 = call "GetNumCamFramesv2.vi"("Digital Waveform Graph"=w1776) -> ("Numeric"=w1777:i32)  [unwired: 10 in]
                    n4737 = local write "Digital Lines Plot"(w1776) -> ()
                    n4738 = case shown="True" w1770 {
                      tunnel: w1769 -> [_ w1790]
                      frame False {
                      }
                      frame True {
                        n4739 = local write "# of frames"(w1790) -> ()
                      }
                    }
                    n4740 = call "waveformsAObuffer.vi"("AO wf in"=w1778, "command"="set") -> ()  [unwired: 1 out]
                    n4741 = call "waveformsDObuffer.vi"("DO wf in"=w1776, "command"="set") -> ()  [unwired: 1 out]
                    n4742 = local write "Total Camera Frames"(w1777) -> ()
                  }
                }
              }
              frame #4 {
                n4743 = local read "finite samples"() -> (w1791:bool)
                n4744 = local read "continuous"() -> (w1792:bool)
                n4745 = local read "wavdet"() -> (w1793:bool)
                n4746 = call "2pparameters.vi"("command"="get") -> ("params out"=w1796:T10)  [unwired: 1 in]
                n4747 = Bundle By Name(cluster=w1796, "finite"=w1791, "cont"=w1792, "wavdet"=w1793) -> (w1794:T10)
                n4748 = call "2pparameters.vi"("Params in"=w1794, "command"="set") -> ()  [unwired: 1 out]
              }
            }
          }
          event "Add settings": Value Change {
            n4749 = event-data() -> ()  [unwired: 1 in, 6 out]
            n4750 = call "wfsettings.vi"("command"="get") -> ("wfsettings out"=w1800:T27)  [unwired: 2 in, 1 out]
            n4751 = in-place {
              n4752 = in-place-cluster #53(w1800) -> ("settings names"=w1805:string[], "settings locations"=w1807:path[])
              n4753 = local read "Setting location"() -> (w1803:path)
              n4754 = local read "Nickname"() -> (w1802:string)
              n4755 = Build Array (concatenate)(w1805, w1802) -> (w1804:string[])
              n4756 = property on="Loaded settings" class="Ring (strict)"("Strings []"=w1804) -> ()  [unwired: 2 in, 2 out]
              n4757 = Build Array (concatenate)(w1807, w1803) -> (w1806:path[])
              n4758 = in-place-cluster #53("settings names"=w1804, "settings locations"=w1806) -> (w1798:T27)
            }
            n4759 = call "wfsettings.vi"("wfsettings in"=w1798, "command"="set") -> ()  [unwired: 1 in, 2 out]
          }
          event "Rem setting": Value Change {
            n4760 = event-data() -> ()  [unwired: 1 in, 6 out]
            n4761 = call "wfsettings.vi"("command"="get") -> ("wfsettings out"=w1810:T27)  [unwired: 2 in, 1 out]
            n4762 = in-place {
              n4763 = in-place-cluster #54(w1810) -> ("settings names"=w1815:string[], "settings locations"=w1813:path[])
              n4764 = property on="Loaded settings" class="Ring (strict)"() -> ("RingText.Text"=w1816:string)  [unwired: 2 in, 2 out]
              n4765 = Search 1D Array(1D array=w1815, element=w1816) -> (index of element=w1817:i32)  [unwired: 1 in]
              n4766 = Delete From Array(array=w1815, index=w1817) -> (array with subset deleted=w1814:string[])  [unwired: 1 in, 1 out]
              n4767 = Delete From Array(array=w1813, index=w1817) -> (array with subset deleted=w1812:path[])  [unwired: 1 in, 1 out]
              n4768 = property on="Loaded settings" class="Ring (strict)"("Strings []"=w1814) -> ()  [unwired: 2 in, 2 out]
              n4769 = in-place-cluster #54("settings names"=w1814, "settings locations"=w1812) -> (w1808:T27)
            }
            n4770 = call "wfsettings.vi"("wfsettings in"=w1808, "command"="set") -> ()  [unwired: 1 in, 2 out]
          }
          event "Update settings": Value Change {
            n4771 = event-data() -> ()  [unwired: 1 in, 6 out]
            n4772 = stacked-sequence {
              frame #0 {
                n4773 = local read "Measurement"() -> (w1818:T4)
                n4774 = case shown="\"Timetrace\"" w1818 {
                  frame "X-Y-t movie", Default {
                    n4775 = local read "avpp"() -> (w1839:i32)
                    n4776 = local read "Angle ref"() -> (w1838:dbl)
                    n4777 = local read "ROI Type"() -> (w1837:u16)
                    n4778 = local read "xpixels ref"() -> (w1834:i32)
                    n4779 = local read "Vx-min ref"() -> (w1833:dbl)
                    n4780 = local read "Vx-max ref"() -> (w1832:dbl)
                    n4781 = local read "ypixels ref"() -> (w1830:i32)
                    n4782 = local read "Vy-min ref"() -> (w1831:dbl)
                    n4783 = local read "Vy-max ref"() -> (w1827:dbl)
                    n4784 = local read "Sampling rate"() -> (w1821:dbl)
                    n4785 = local read "finite samples"() -> (w1822:bool)
                    n4786 = local read "continuous"() -> (w1825:bool)
                    n4787 = local read "wavdet"() -> (w1826:bool)
